vi "Stop Stream and Reset RX FIFO.vi"(8 "error in (no error)":errorcluster, 10 "2 USRPs?":bool[](array[boolean]), 11 "Refnum in":refnum<k20>[](array[refnum])) -> (0 "error out":errorcluster, 3 "Refnum out":refnum<k20>[](array[refnum]))   [LabVIEW 2016]
uses:
  <instrlib>/_niInstr/Streaming/v1/Host/niInstr Streaming v1 Host.lvlib
  6592R/SubVIs/Aurora Stream (NI 6592R) (Host).lvlib
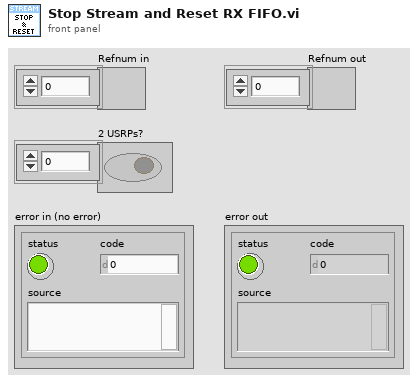
[diagram p1: front panel]
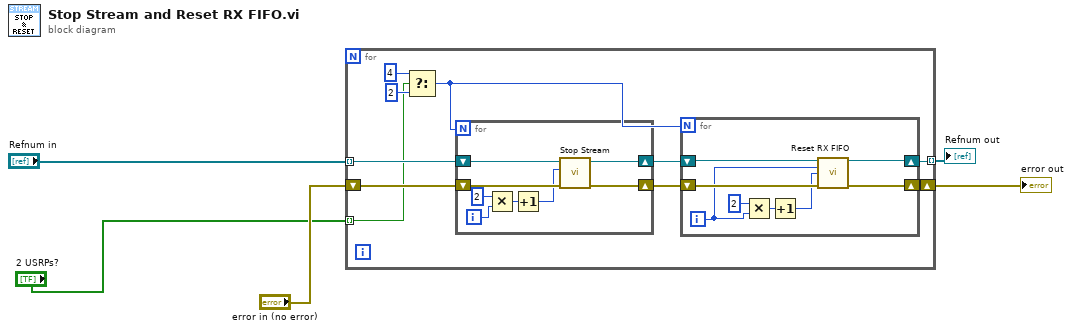
[diagram p0: block diagram]
diagram:
  n1 = for {
    tunnel: "Refnum in" -> [w14] mode=indexing
    tunnel: [w7] -> w2 mode=indexing
    shift-right: [w8] -> w3
    shift-left: "error in (no error)" -> [w15]
    tunnel: "2 USRPs?" -> [w11] mode=indexing
    n2 = Select(t=4, s=w11, f=2) -> (s? t:f=w6:i32)
    n3 = for {
      N: w6 -> [_]
      shift-right: [w29] -> w9
      shift-left: w14 -> [w30]
      shift-right: [w28] -> w10
      shift-left: w15 -> [w31]
      i -> [w25]
      n4 = Multiply(x=2, y=w25) -> (x*y=w26:i32)
      n5 = Increment(x=w26) -> (x+1=w24:i32)
      n6 = call <instrlib>:"Stop Stream.vi"("error in (no error)"=w31, "stream index"=w24, "refnum in"=w30) -> ("error out"=w28:errorcluster, "refnum out"=w29:refnum<k20>)  [unwired: 5 in, 2 out]
    }
    n7 = for {
      N: w6 -> [_]
      shift-right: [w21] -> w7
      shift-left: w9 -> [w22]
      shift-right: [w20] -> w8
      shift-left: w10 -> [w23]
      i -> [w17]
      n8 = Multiply(x=2, y=w17) -> (x*y=w19:i32)
      n9 = Increment(x=w19) -> (x+1=w16:i32)
      n10 = call "Reset RX FIFO.vi"("Refnum in"=w22, "Port"=w17, "stream index"=w16, "error in"=w23) -> ("Refnum out"=w21:refnum<k20>, "error out"=w20:errorcluster)  [unwired: 10 in]
    }
  }
  "error out" <- w3
  "Refnum out" <- w2
